vi "Waveform, Trim Head.vi"(0 "error in":errorcluster, 1 "lower limit (-0.05)":dbl=-0.05, 2 "upper limit (0.05)":dbl=0.05, 3 "waveform":waveform(dbl)={"t0"=timestamp(3476124940.313 s since 1904-01-01), "dt"=1e-08, "Y"=[], "attributes"=variant("Average Size"=variant(dbl 15.0), "Frequency (Hz)"=variant(dbl 2001.2998047407427), "Interphase Delay (us)"=variant(dbl 16.2725), "Number of Samples"=variant(dbl 400000.0), "Process Timestamp"=variant(dbl 3476272955.921875), "Recvy Amp (V)"=variant(dbl 2.524589445147007), "Recvy Amp (mA)"=variant(dbl 5.049178890294014), "Recvy Duty Factor"=variant(dbl 0.023418514965706478), "Recvy Frequency (Hz)"=variant(dbl 2001.4010193262206), "Recvy Period (us)"=variant(dbl 499.6499903535843), "Recvy Pulse Width (us)"=variant(dbl 11.701060776710511), "Recvy Trigger (s)"=variant(dbl 0.00041576), "Resistance (ohms)"=variant(dbl 500.0), "Sample Frequency (MHz)"=variant(dbl 100.0), "Stim Amp (V)"=variant(dbl -2.427167122033602), "Stim Amp (mA)"=variant(dbl -4.8543342440672035), "Stim Duty Factor"=variant(dbl 0.023054309749159837), "Stim Frequency (Hz)"=variant(dbl 2001.1985901552648), "Stim Period (us)"=variant(dbl 499.70053193092355), "Stim Pulse Width (us)"=variant(dbl 11.520250844955445), "Stim Trigger (s)"=variant(dbl 0.00038793000000000003), "dt (us)"=variant(dbl 0.01))}, 4 "interval (250 us)":dbl=250.0 format="%.1f") -> (7 "error out":errorcluster, 9 "trim (ms)":dbl=0.10603 format="%.3f", 10 "waveform out":waveform(dbl)={"t0"=timestamp(-9593182799.687 s since 1904-01-01), "dt"=nan, "Y"=[], "attributes"=variant("Average Size"=variant(dbl 15.0), "Frequency (Hz)"=variant(dbl 2001.2998047407427), "Interphase Delay (us)"=variant(dbl 16.2725), "Number of Samples"=variant(dbl 400000.0), "Process Timestamp"=variant(dbl 3476272955.921875), "Recvy Amp (V)"=variant(dbl 2.524589445147007), "Recvy Amp (mA)"=variant(dbl 5.049178890294014), "Recvy Duty Factor"=variant(dbl 0.023418514965706478), "Recvy Frequency (Hz)"=variant(dbl 2001.4010193262206), "Recvy Period (us)"=variant(dbl 499.6499903535843), "Recvy Pulse Width (us)"=variant(dbl 11.701060776710511), "Recvy Trigger (s)"=variant(dbl 0.00041576), "Resistance (ohms)"=variant(dbl 500.0), "Sample Frequency (MHz)"=variant(dbl 100.0), "Stim Amp (V)"=variant(dbl -2.427167122033602), "Stim Amp (mA)"=variant(dbl -4.8543342440672035), "Stim Duty Factor"=variant(dbl 0.023054309749159837), "Stim Frequency (Hz)"=variant(dbl 2001.1985901552648), "Stim Period (us)"=variant(dbl 499.70053193092355), "Stim Pulse Width (us)"=variant(dbl 11.520250844955445), "Stim Trigger (s)"=variant(dbl 0.00038793000000000003), "dt (us)"=variant(dbl 0.01))})   [LabVIEW 2010]
doc: "This function searches for the first contiguous interval of data in a waveform that is within the upper and lower limits. If the filter criteria is met, all data from the start of the waveform to the end of the data set is trimmed (removed)."
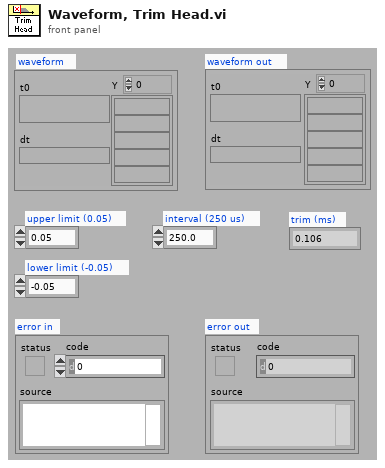
[diagram p1: front panel]
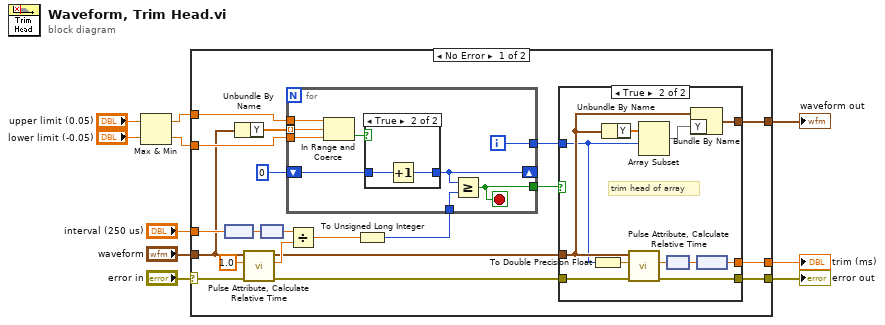
[diagram p0: block diagram]
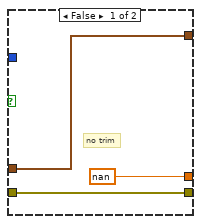
[diagram p2: hidden frame]
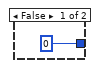
[diagram p3: hidden frame]
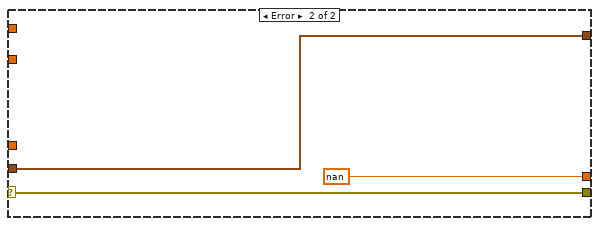
[diagram p4: hidden frame]
diagram:
  n1 = Max & Min(x="upper limit (0.05)", y="lower limit (-0.05)") -> (max(x,y)=w1:dbl, min(x,y)=w3:dbl)
  n2 = case shown="No Error" "error in" {
    selector: "error in" -> [w23 w59]
    tunnel: w1 -> [w30 _]
    tunnel: w3 -> [w29 _]
    tunnel: "waveform" -> [w14 w58]
    tunnel: [w26 w58] -> w8
    tunnel: [w25 w59] -> w9
    tunnel: "interval (250 us)" -> [w17 _]
    tunnel: [w24 nan] -> w5
    frame No Error {
      n3 = node(w17) -> (w19:dbl[unit])
      n4 = Unbundle By Name(w14) -> ("Y"=w27:dbl[])
      n5 = call "Pulse Attribute, Calculate Relative Time.vi"("error in"=w23, "index"=1.0, "waveform"=w14) -> ("error out"=w22:errorcluster, "relative time (s)"=w20:dbl, "waveform dup"=w13:waveform(dbl))  [unwired: 4 in]
      n6 = node(w19) -> (w18:dbl)
      n7 = Divide(x=w18, y=w20) -> (x/y=w16:dbl)
      n8 = To Unsigned Long Integer(number=w16) -> (unsigned 32bit integer=w15:u32)
      n9 = for {
        tunnel: w27 -> [w51] mode=indexing
        tunnel: w29 -> [w50]
        tunnel: w30 -> [w52]
        shift-right: [w48] -> _
        shift-left: u32 0 -> [w53]
        tunnel: [w47] -> w12
        tunnel: [w45] -> w11
        tunnel: w15 -> [w46]
        i -> [w47]
        stop <- w45 stop-if-true
        n10 = In Range and Coerce(upper limit=w52, x=w51, lower limit=w50) -> (In Range?=w49:bool)  [unwired: 1 out]
        n11 = case shown="True" w49 {
          tunnel: [u32 0 w55] -> w48
          tunnel: w53 -> [_ w56]
          frame False {
          }
          frame True {
            n12 = Increment(x=w56) -> (x+1=w55:u32)
          }
        }
        n13 = Greater Or Equal?(x=w48, y=w46) -> (x >= y?=w45:bool)
      }
      n14 = case shown="True" w11 {
        tunnel: [w33 w44] -> w26
        tunnel: [w32 w43] -> w25
        tunnel: [nan w39] -> w24
        tunnel: w22 -> [w32 w38]
        tunnel: w13 -> [w33 w35]
        tunnel: w12 -> [_ w34]
        frame False {
          # "no trim"
        }
        frame True {
          # "trim head of array"
          n15 = To Double Precision Float(number=w34) -> (double precision float=w41:dbl)
          n16 = Unbundle By Name(w35) -> ("Y"=w36:dbl[])
          n17 = call "Pulse Attribute, Calculate Relative Time.vi"("error in"=w38, "index"=w41, "waveform"=w35) -> ("error out"=w43:errorcluster, "relative time (s)"=w42:dbl)  [unwired: 4 in, 1 out]
          n18 = Array Subset(array=w36, index=w34) -> (w37:dbl[])  [unwired: 1 in]
          n19 = node(w42) -> (w40:dbl[unit])
          n20 = Bundle By Name(cluster=w35, "Y"=w37) -> (w44:waveform(dbl))
          n21 = node(w40) -> (w39:dbl)
        }
      }
    }
    frame Error {
    }
  }
  "waveform out" <- w8
  "error out" <- w9
  "trim (ms)" <- w5
